vi "Get phases.vi"(8 "error in (no error)":errorcluster, 11 "ImagingModeSPIM in":refnum<class "ImagingModeSPIM.lvclass">) -> (0 "error out":errorcluster, 3 "ImagingModeSPIM out":refnum<class "ImagingModeSPIM.lvclass">)   [LabVIEW 2012, in "ImagingModeSPIM.lvclass"]
uses:
  ImagingModeSPIM.lvclass
  ImagingModeSPIM.lvclass/ImagingModeSPIM.ctl
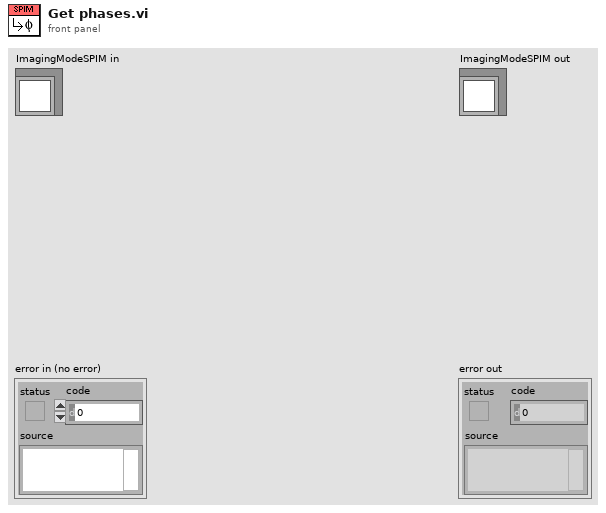
[diagram p1: front panel]
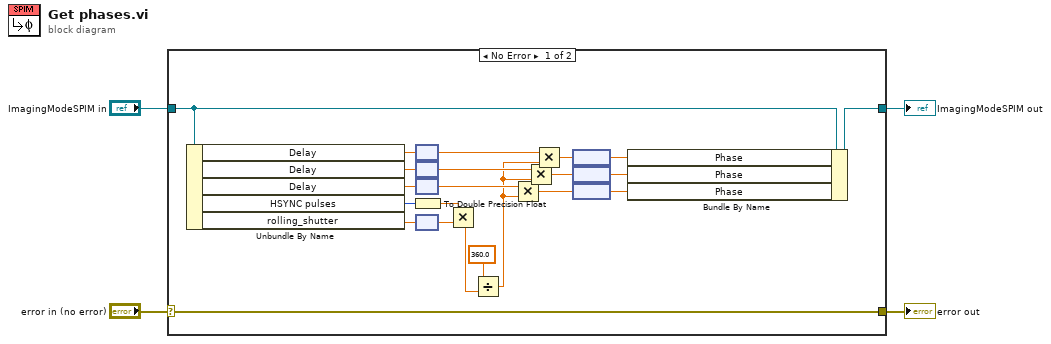
[diagram p0: block diagram]
diagram:
  n1 = case shown="No Error" "error in (no error)" {
    selector: "error in (no error)" -> [w26 w28]
    tunnel: [w26 w28] -> w3
    tunnel: [w24 w27] -> w1
    tunnel: "ImagingModeSPIM in" -> [w25 w27]
    frame No Error {
      n2 = Unbundle By Name(w25) -> ("Delay"=w17:dbl[unit], "Delay"=w18:dbl[unit], "Delay"=w19:dbl[unit], "HSYNC pulses"=w23:i32, "rolling_shutter"=w22:dbl[unit])
      n3 = To Double Precision Float(number=w23) -> (double precision float=w21:dbl)
      n4 = node(w17) -> (w14:dbl)
      n5 = node(w18) -> (w13:dbl)
      n6 = node(w19) -> (w12:dbl)
      n7 = node(w22) -> (w20:dbl)
      n8 = Multiply(x=w21, y=w20) -> (x*y=w15:dbl)
      n9 = Divide(x=360.0 ("y"), y=w15) -> (x/y=w11:dbl)
      n10 = Multiply(x=w12, y=w11) -> (x*y=w7:dbl)
      n11 = Multiply(x=w13, y=w11) -> (x*y=w8:dbl)
      n12 = Multiply(x=w14, y=w11) -> (x*y=w10:dbl)
      n13 = node(w10) -> (w9:dbl[unit])
      n14 = node(w8) -> (w6:dbl[unit])
      n15 = node(w7) -> (w5:dbl[unit])
      n16 = Bundle By Name(cluster=w25, "Phase"=w9, "Phase"=w6, "Phase"=w5) -> (w24:refnum<class "ImagingModeSPIM.lvclass">)
    }
    frame Error {
    }
  }
  "error out" <- w3
  "ImagingModeSPIM out" <- w1
